vi "rsscope_core_global.vi"() -> ()   [LabVIEW 2018] (continued)
Name"="PCIe Trigger ERRC Unknown Packet", "Data Type"=3, "Command"="TRIG{Trigger}:PCIE:ERRC:UKNP", "Access"=2, "Range Table"="", "Read Callback"="", "Write Callback"="", "Supported Models"="RTO|RTP", "Instrument Options"="K72", "Flags"=0, "Help"="Enables triggering on an unknown packet.\n\nAvailable Repeated Capabilities:\nTrigger: TrigA, TrigB, TrigR\r\n\nRemote-control command(s):\nTRIGger<m>:PCIE:ERRC:UKNP"}, {"Level"=2, "Class Only"=TRUE, "Identifier"="", "Descriptive Name"="EbTb", "Data Type"=0, "Command"="", "Access"=0, "Range Table"="", "Read Callback"="", "Write Callback"="", "Supported Models"="", "Instrument Options"="", "Flags"=0, "Help"="The trigger suffix <m> is always 1 and can be omitted. It selects the trigger event: Only\nthe A-trigger is available for triggering on serial buses."}, {"Level"=3, "Class Only"=FALSE, "Identifier"="RSSCOPE_ATTR_EBTB_TRIGGER_TYPE", "Descriptive Name"="EbTb Trigger Type", "Data Type"=0, "Command"="TRIG{Trigger}:EBTB:TYPE", "Access"=2, "Range Table"="RsScope_rngEbTbTriggerType", "Read Callback"="", "Write Callback"="", "Supported Models"="", "Instrument Options"="", "Flags"=0, "Help"="Selects the type of condition to be triggered on. You can trigger on a certain symbol or enable a specific error condition.\n\nAvailable Repeated Capabilities:\nTrigger: TrigA, TrigB, TrigR\r\n\nRemote-control command(s):\nTRIGger<m>:EBTB:TYPE"}, {"Level"=3, "Class Only"=FALSE, "Identifier"="RSSCOPE_ATTR_EBTB_TRIGGER_CONDITION_TYPE", "Descriptive Name"="EbTb Trigger Condition Type", "Data Type"=0, "Command"="TRIG{Trigger}:EBTB:STYP", "Access"=2, "Range Table"="RsScope_rngTriggerConditionType", "Read Callback"="", "Write Callback"="", "Supported Models"="", "Instrument Options"="", "Flags"=0, "Help"="Selects the type of condition to be triggered on for 8b10b.\n\nAvailable Repeated Capabilities:\nTrigger: TrigA, TrigB, TrigR\r\n\nRemote-control command(s):\nTRIGger<m>:EBTB:STYPe"}, {"Level"=3, "Class Only"=FALSE, "Identifier"="RSSCOPE_ATTR_EBTB_TRIGGER_DISPARITY_ERROR", "Descriptive Name"="EbTb Trigger Disparity Error", "Data Type"=3, "Command"="TRIG{Trigger}:EBTB:DISP", "Access"=2, "Range Table"="", "Read Callback"="", "Write Callback"="", "Supported Models"="", "Instrument Options"="K52", "Flags"=0, "Help"="Defines, if a trigger on a disparity error is activated or not.\n\nAvailable Repeated Capabilities:\nTrigger: TrigA, TrigB, TrigR\r\n\nRemote-control command(s):\nTRIGger<m>:EBTB:DISParityerr"}, {"Level"=3, "Class Only"=FALSE, "Identifier"="RSSCOPE_ATTR_EBTB_TRIGGER_DATA_CHARACTER", "Descriptive Name"="EbTb Trigger Data Character", "Data Type"=0, "Command"="TRIG{Trigger}:EBTB:SYMT", "Access"=2, "Range Table"="RsScope_rngEbTbTriggerDataCharacter", "Read Callback"="", "Write Callback"="", "Supported Models"="", "Instrument Options"="K52", "Flags"=0, "Help"="Selects the data character (Dx.y) or control character to be triggered on. You can specify the value of the data character to be triggered on with RSSCOPE_ATTR_EBTB_TRIGGER_DX_SYMBOL and RSSCOPE_ATTR_EBTB_TRIGGER_DY_SYMBOL.\n\nAvailable Repeated Capabilities:\nTrigger: TrigA, TrigB, TrigR\r\n\nRemote-control command(s):\nTRIGger<m>:EBTB:SYMType"}, {"Level"=3, "Class Only"=FALSE, "Identifier"="RSSCOPE_ATTR_EBTB_TRIGGER_DX_SYMBOL", "Descriptive Name"="EbTb Trigger DX Symbol", "Data Type"=0, "Command"="TRIG{Trigger}:EBTB:DX", "Access"=2, "Range Table"="RsScope_rngEbTbTriggerDXSymbol", "Read Callback"="", "Write Callback"="", "Supported Models"="", "Instrument Options"="K52", "Flags"=0, "Help"="Sets thex value of the data character Dx.y to be triggered on.\n\nAvailable Repeated Capabilities:\nTrigger: TrigA, TrigB, TrigR\r\n\nRemote-control command(s):\nTRIGger<m>:EBTB:DX"}, {"Level"=3, "Class Only"=FALSE, "Identifier"="RSSCOPE_ATTR_EBTB_TRIGGER_DY_SYMBOL", "Descriptive Name"="EbTb Trigger DY Symbol", "Data Type"=0, "Command"="TRIG{Trigger}:EBTB:DY", "Access"=2, "Range Table"="RsScope_rngEbTbTriggerDYSymbol", "Read Callback"="", "Write Callback"="", "Supported Models"="", "Instrument Options"="K52", "Flags"=0, "Help"="Sets the y value of the data character Dx.y to be triggered on.\n\nAvailable Repeated Capabilities:\nTrigger: TrigA, TrigB, TrigR\r\n\nRemote-control command(s):\nTRIGger<m>:EBTB:DY"}, {"Level"=3, "Class Only"=FALSE, "Identifier"="RSSCOPE_ATTR_EBTB_TRIGGER_SYMBOL_FORMAT", "Descriptive Name"="EbTb Trigger Symbol Format", "Data Type"=0, "Command"="TRIG{Trigger}:EBTB:SYMF", "Access"=2, "Range Table"="RsScope_rngEbTbSymbTrgSymbolFormat", "Read Callback"="", "Write Callback"="", "Supported Models"="", "Instrument Options"="K52", "Flags"=0, "Help"="Selects the format of the symbol to be triggerd on, if TRIGger<m>:EBTB:SSTYpe is set to SYMBol.\n\nAvailable Repeated Capabilities:\nTrigger: TrigA, TrigB, TrigR\r\n\nRemote-control command(s):\nTRIGger<m>:EBTB:SYMFormat"}, {"Level"=3, "Class Only"=FALSE, "Identifier"="RSSCOPE_ATTR_EBTB_TRIGGER_EB_PATTERN", "Descriptive Name"="EbTb Trigger EB Pattern", "Data Type"=2, "Command"="TRIG{Trigger}:EBTB:EBPA", "Access"=2, "Range Table"="", "Read Callback"="", "Write Callback"="", "Supported Models"="", "Instrument Options"="K52", "Flags"=0, "Help"="Sets the 8-bit pattern to be triggered on, if TRIGger<m>:EBTB:SYMFormat is set to EB.\n\nAvailable Repeated Capabilities:\nTrigger: TrigA, TrigB, TrigR\r\n\nRemote-control command(s):\nTRIGger<m>:EBTB:EBPA"}, {"Level"=3, "Class Only"=FALSE, "Identifier"="RSSCOPE_ATTR_EBTB_TRIGGER_TB_PATTERN", "Descriptive Name"="EbTb Trigger TB Pattern", "Data Type"=2, "Command"="TRIG{Trigger}:EBTB:TBPA", "Access"=2, "Range Table"="", "Read Callback"="", "Write Callback"="", "Supported Models"="", "Instrument Options"="K52", "Flags"=0, "Help"="Sets the 10-bit pattern to be triggered on, if TRIGger<m>:EBTB:SYMFormat is set to TB.\n\nAvailable Repeated Capabilities:\nTrigger: TrigA, TrigB, TrigR\r\n\nRemote-control command(s):\nTRIGger<m>:EBTB:TBPA"}, {"Level"=3, "Class Only"=FALSE, "Identifier"="RSSCOPE_ATTR_EBTB_TRIGGER_GLITCH_ERROR", "Descriptive Name"="EbTb Trigger Glitch Error", "Data Type"=3, "Command"="TRIG{Trigger}:EBTB:GLIT", "Access"=2, "Range Table"="", "Read Callback"="", "Write Callback"="", "Supported Models"="", "Instrument Options"="K52", "Flags"=0, "Help"="Defines, if a trigger on a glitch error is activated or not.\n\nAvailable Repeated Capabilities:\nTrigger: TrigA, TrigB, TrigR\r\n\nRemote-control command(s):\nTRIGger<m>:EBTB:GLITcherror"}, {"Level"=3, "Class Only"=FALSE, "Identifier"="RSSCOPE_ATTR_EBTB_TRIGGER_SYMBOL_TYPE", "Descriptive Name"="EbTb Trigger Symbol Type", "Data Type"=0, "Command"="TRIG{Trigger}:EBTB:SSTY", "Access"=2, "Range Table"="RsScope_rngEbTbTriggerSymbolType", "Read Callback"="", "Write Callback"="", "Supported Models"="", "Instrument Options"="K52", "Flags"=0, "Help"="Selects the symbol type to be triggered on. You can select a single symbol or an expression (defined series of symbols).\n\nAvailable Repeated Capabilities:\nTrigger: TrigA, TrigB, TrigR\r\n\nRemote-control command(s):\nTRIGger<m>:EBTB:SSTYpe"}, {"Level"=3, "Class Only"=FALSE, "Identifier"="RSSCOPE_ATTR_EBTB_TRIGGER_SYMBOL_EXPRESSION", "Descriptive Name"="EbTb Trigger Symbol Expression", "Data Type"=2, "Command"="TRIG{Trigger}:EBTB:SYME", "Access"=2, "Range Table"="", "Read Callback"="", "Write Callback"="", "Supported Models"="", "Instrument Options"="K52", "Flags"=0, "Help"="Selects the format of the symbol to be triggered on, if TRIGger<m>:EBTB:SSTYpe is set to EXPRession.\n\nAvailable Repeated Capabilities:\nTrigger: TrigA, TrigB, TrigR\r\n\nRemote-control command(s):\nTRIGger<m>:EBTB:SYME"}, {"Level"=3, "Class Only"=FALSE, "Identifier"="RSSCOPE_ATTR_EBTB_TRIGGER_UNKNOWN_ERROR", "Descriptive Name"="EbTb Trigger Unknown Error", "Data Type"=3, "Command"="TRIG{Trigger}:EBTB:UNK", "Access"=2, "Range Table"="", "Read Callback"="", "Write Callback"="", "Supported Models"="", "Instrument Options"="K52", "Flags"=0, "Help"="Defines, if a trigger on a unknown symbol error is activated or not.\n\nAvailable Repeated Capabilities:\nTrigger: TrigA, TrigB, TrigR\r\n\nRemote-control command(s):\nTRIGger<m>:EBTB:UNK"}, {"Level"=2, "Class Only"=TRUE, "Identifier"="", "Descriptive Name"="100BASET1", "Data Type"=0, "Command"="", "Access"=0, "Range Table"="", "Read Callback"="", "Write Callback"="", "Supported Models"="", "Instrument Options"="", "Flags"=0, "Help"="Configures 100BASE-T1 trigger settings.\n\nAttributes in this class require option R&S RTO-K57."}, {"Level"=3, "Class Only"=FALSE, "Identifier"="RSSCOPE_ATTR_100BASE_T1_TRIGGER_TYPE", "Descriptive Name"="100BASE-T1 Trigger Type", "Data Type"=0, "Command"="TRIG{Trigger}:HBTO:TYPE", "Access"=2, "Range Table"="RsScope_rng100BASE_T1FrameType", "Read Callback"="", "Write Callback"="", "Supported Models"="", "Instrument Options"="K57", "Flags"=0, "Help"="Selects the type of frame to be triggered on.\n\nAvailable Repeated Capabilities:\nTrigger: TrigA, TrigB, TrigR\r\n\nRemote-control command(s):\nTRIGger<m>:HBTO:TYPE"}, {"Level"=3, "Class Only"=FALSE, "Identifier"="RSSCOPE_ATTR_100BASE_T1_TRIGGER_DESTINATION_ADDRESS_CONDITION", "Descriptive Name"="100BASE-T1 Trigger Destination Address Condition", "Data Type"=0, "Command"="TRIG{Trigger}:HBTO:DADD:COND", "Access"=2, "Range Table"="rsscope_rngProtocolTriggerCondition", "Read Callback"="", "Write Callback"="", "Supported Models"="", "Instrument Options"="K57", "Flags"=0, "Help"="Sets the condition for the destination address. You can define an exact value or a value range.\n\nAvailable Repeated Capabilities:\nTrigger: TrigA, TrigB, TrigR\r\n\nRemote-control command(s):\nTRIGger<m>:HBTO:DADDress:CONDition"}, {"Level"=3, "Class Only"=FALSE, "Identifier"="RSSCOPE_ATTR_100BASE_T1_TRIGGER_DESTINATION_ADDRESS_MIN", "Descriptive Name"="100BASE-T1 Trigger Destination Address Min", "Data Type"=2, "Command"="TRIG{Trigger}:HBTO:DADD:MIN", "Access"=2, "Range Table"="", "Read Callback"="", "Write Callback"="", "Supported Models"="", "Instrument Options"="K57", "Flags"=0, "Help"="Specifies the destination address bit pattern, or sets the start value of a pattern range.\n\nAvailable Repeated Capabilities:\nTrigger: TrigA, TrigB, TrigR\r\n\nRemote-control command(s):\nTRIGger<m>:HBTO:DADDress:MIN"}, {"Level"=3, "Class Only"=FALSE, "Identifier"="RSSCOPE_ATTR_100BASE_T1_TRIGGER_DESTINATION_ADDRESS_MAX", "Descriptive Name"="100BASE-T1 Trigger Destination Address Max", "Data Type"=2, "Command"="TRIG{Trigger}:HBTO:DADD:MAX", "Access"=2, "Range Table"="", "Read Callback"="", "Write Callback"="", "Supported Models"="", "Instrument Options"="K57", "Flags"=0, "Help"="Sets the end value of the destination address range if the corresponding condition is set to In Range or Out Of Range.\n\nAvailable Repeated Capabilities:\nTrigger: TrigA, TrigB, TrigR\r\n\nRemote-control command(s):\nTRIGger<m>:HBTO:DADDress:MAX"}, {"Level"=3, "Class Only"=FALSE, "Identifier"="RSSCOPE_ATTR_100BASE_T1_TRIGGER_SOURCE_ADDRESS_CONDITION", "Descriptive Name"="100BASE-T1 Trigger Source Address Condition", "Data Type"=0, "Command"="TRIG{Trigger}:HBTO:SADD:COND", "Access"=2, "Range Table"="rsscope_rngProtocolTriggerCondition", "Read Callback"="", "Write Callback"="", "Supported Models"="", "Instrument Options"="K57", "Flags"=0, "Help"="Sets the condition for the source address. You can define an exact value or a value range.\n\nAvailable Repeated Capabilities:\nTrigger: TrigA, TrigB, TrigR\r\n\nRemote-control command(s):\nTRIGger<m>:HBTO:SADDress:CONDition"}, {"Level"=3, "Class Only"=FALSE, "Identifier"="RSSCOPE_ATTR_100BASE_T1_TRIGGER_SOURCE_ADDRESS_MIN", "Descriptive Name"="100BASE-T1 Trigger Source Address Min", "Data Type"=2, "Command"="TRIG{Trigger}:HBTO:SADD:MIN", "Access"=2, "Range Table"="", "Read Callback"="", "Write Callback"="", "Supported Models"="", "Instrument Options"="K57", "Flags"=0, "Help"="Specifies the source address bit pattern, or sets the start value of a pattern range.\n\nAvailable Repeated Capabilities:\nTrigger: TrigA, TrigB, TrigR\r\n\nRemote-control command(s):\nTRIGger<m>:HBTO:SADDress:MIN"}, {"Level"=3, "Class Only"=FALSE, "Identifier"="RSSCOPE_ATTR_100BASE_T1_TRIGGER_SOURCE_ADDRESS_MAX", "Descriptive Name"="100BASE-T1 Trigger Source Address Max", "Data Type"=2, "Command"="TRIG{Trigger}:HBTO:SADD:MAX", "Access"=2, "Range Table"="", "Read Callback"="", "Write Callback"="", "Supported Models"="", "Instrument Options"="K57", "Flags"=0, "Help"="Sets the end value of the source address range if the corresponding condition is set to In Range or Out Of Range.\n\nAvailable Repeated Capabilities:\nTrigger: TrigA, TrigB, TrigR\r\n\nRemote-control command(s):\nTRIGger<m>:HBTO:SADDress:MAX"}, {"Level"=3, "Class Only"=FALSE, "Identifier"="RSSCOPE_ATTR_100BASE_T1_TRIGGER_TYPE_LENGTH_CONDITION", "Descriptive Name"="100BASE-T1 Trigger Type Length Condition", "Data Type"=0, "Command"="TRIG{Trigger}:HBTO:LENG:COND", "Access"=2, "Range Table"="rsscope_rngProtocolTriggerCondition", "Read Callback"="", "Write Callback"="", "Supported Models"="", "Instrument Options"="K57", "Flags"=0, "Help"="Sets the condition for the length / type. You can define an exact value or a value range.\n\nAvailable Repeated Capabilities:\nTrigger: TrigA, TrigB, TrigR\r\n\nRemote-control command(s):\nTRIGger<m>:HBTO:LENGth:CONDition"}, {"Level"=3, "Class Only"=FALSE, "Identifier"="RSSCOPE_ATTR_100BASE_T1_TRIGGER_TYPE_LENGTH_MIN", "Descriptive Name"="100BASE-T1 Trigger Type Length Min", "Data Type"=2, "Command"="TRIG{Trigger}:HBTO:LENG:MIN", "Access"=2, "Range Table"="", "Read Callback"="", "Write Callback"="", "Supported Models"="", "Instrument Options"="", "Flags"=0, "Help"="Specifies the length / type bit pattern, or sets the start value of a pattern range.\n\nAvailable Repeated Capabilities:\nTrigger: TrigA, TrigB, TrigR\r\n\nRemote-control command(s):\nTRIGger<m>:HBTO:LENGth:MIN"}, {"Level"=3, "Class Only"=FALSE, "Identifier"="RSSCOPE_ATTR_100BASE_T1_TRIGGER_TYPE_LENGTH_MAX", "Descriptive Name"="100BASE-T1 Trigger Type Length Max", "Data Type"=2, "Command"="TRIG{Trigger}:HBTO:LENG:MAX", "Access"=2, "Range Table"="", "Read Callback"="", "Write Callback"="", "Supported Models"="", "Instrument Options"="K57", "Flags"=0, "Help"="Sets the end value of the length / type range if the corresponding condition is set to In Range or Out Of Range.\n\nAvailable Repeated Capabilities:\nTrigger: TrigA, TrigB, TrigR\r\n\nRemote-control command(s):\nTRIGger<m>:HBTO:LENGth:MAX"}, {"Level"=3, "Class Only"=FALSE, "Identifier"="RSSCOPE_ATTR_100BASE_T1_TRIGGER_CRC_CONDITION", "Descriptive Name"="100BASE-T1 Trigger CRC Condition", "Data Type"=0, "Command"="TRIG{Trigger}:HBTO:CRC:COND", "Access"=2, "Range Table"="rsscope_rngProtocolTriggerCondition", "Read Callback"="", "Write Callback"="", "Supported Models"="", "Instrument Options"="K57", "Flags"=0, "Help"="Sets the condition for the frame check. You can define an exact value or a value range.\n\nAvailable Repeated Capabilities:\nTrigger: TrigA, TrigB, TrigR\r\n\nRemote-control command(s):\nTRIGger<m>:HBTO:CRC:CONDition"}, {"Level"=3, "Class Only"=FALSE, "Identifier"="RSSCOPE_ATTR_100BASE_T1_TRIGGER_CRC_MIN", "Descriptive Name"="100BASE-T1 Trigger CRC Min", "Data Type"=2, "Command"="TRIG{Trigger}:HBTO:CRC:MIN", "Access"=2, "Range Table"="", "Read Callback"="", "Write Callback"="", "Supported Models"="", "Instrument Options"="K57", "Flags"=0, "Help"="Specifies the frame check bit pattern, or sets the start value of a pattern range.\n\nAvailable Repeated Capabilities:\nTrigger: TrigA, TrigB, TrigR\r\n\nRemote-control command(s):\nTRIGger<m>:HBTO:CRC:MIN"}, {"Level"=3, "Class Only"=FALSE, "Identifier"="RSSCOPE_ATTR_100BASE_T1_TRIGGER_CRC_MAX", "Descriptive Name"="100BASE-T1 Trigger CRC Max", "Data Type"=2, "Command"="TRIG{Trigger}:HBTO:CRC:MAX", "Access"=2, "Range Table"="", "Read Callback"="", "Write Callback"="", "Supported Models"="", "Instrument Options"="K57", "Flags"=0, "Help"="Sets the end value of the frame check range if the corresponding condition is set to In Range or Out Of Range.\n\nAvailable Repeated Capabilities:\nTrigger: TrigA, TrigB, TrigR\r\n\nRemote-control command(s):\nTRIGger<m>:HBTO:CRC:MAX"}, {"Level"=3, "Class Only"=FALSE, "Identifier"="RSSCOPE_ATTR_100BASE_T1_TRIGGER_DATA_CONDITION", "Descriptive Name"="100BASE-T1 Trigger Data Condition", "Data Type"=0, "Command"="TRIG{Trigger}:HBTO:DATA:DCON", "Access"=2, "Range Table"="rsscope_rngProtocolTriggerCondition", "Read Callback"="", "Write Callback"="", "Supported Models"="", "Instrument Options"="K57", "Flags"=0, "Help"="Sets the condition for the data. You can define an exact value or a value range.\n\nAvailable Repeated Capabilities:\nTrigger: TrigA, TrigB, TrigR\r\n\nRemote-control command(s):\nTRIGger<m>:HBTO:DATA:DCONdition"}, {"Level"=3, "Class Only"=FALSE, "Identifier"="RSSCOPE_ATTR_100BASE_T1_TRIGGER_DATA_MIN", "Descriptive Name"="100BASE-T1 Trigger Data Min", "Data Type"=2, "Command"="TRIG{Trigger}:HBTO:DATA:DMIN", "Access"=2, "Range Table"="", "Read Callback"="", "Write Callback"="", "Supported Models"="", "Instrument Options"="K57", "Flags"=0, "Help"="Specifies the data bit pattern, or sets the start value of a pattern range.\n\nAvailable Repeated Capabilities:\nTrigger: TrigA, TrigB, TrigR\r\n\nRemote-control command(s):\nTRIGger<m>:HBTO:DATA:DMIN"}, {"Level"=3, "Class Only"=FALSE, "Identifier"="RSSCOPE_ATTR_100BASE_T1_TRIGGER_DATA_MAX", "Descriptive Name"="100BASE-T1 Trigger Data Max", "Data Type"=2, "Command"="TRIG{Trigger}:HBTO:DATA:DMAX", "Access"=2, "Range Table"="", "Read Callback"="", "Write Callback"="", "Supported Models"="", "Instrument Options"="K57", "Flags"=0, "Help"="Sets the end value of the data range if the corresponding condition is set to In Range or Out Of Range.\n\nAvailable Repeated Capabilities:\nTrigger: TrigA, TrigB, TrigR\r\n\nRemote-control command(s):\nTRIGger<m>:HBTO:DATA:DMAX"}, {"Level"=3, "Class Only"=FALSE, "Identifier"="RSSCOPE_ATTR_100BASE_T1_TRIGGER_INDEX_CONDITION", "Descriptive Name"="100BASE-T1 Trigger Index Condition", "Data Type"=0, "Command"="TRIG{Trigger}:HBTO:DATA:ICON", "Access"=2, "Range Table"="rsscope_rngProtocolTriggerCondition", "Read Callback"="", "Write Callback"="", "Supported Models"="", "Instrument Options"="K57", "Flags"=0, "Help"="Sets the condition for the index. You can define an exact value or a value range.\n\nAvailable Repeated Capabilities:\nTrigger: TrigA, TrigB, TrigR\r\n\nRemote-control command(s):\nTRIGger<m>:HBTO:DATA:ICONdition"}, {"Level"=3, "Class Only"=FALSE, "Identifier"="RSSCOPE_ATTR_100BASE_T1_TRIGGER_INDEX_MIN", "Descriptive Name"="100BASE-T1 Trigger Index Min", "Data Type"=0, "Command"="TRIG{Trigger}:HBTO:DATA:IMIN", "Access"=2, "Range Table"="RsScope_rng100BASE_T1TriggerIndex", "Read Callback"="", "Write Callback"="", "Supported Models"="", "Instrument Options"="K57", "Flags"=0, "Help"="Specifies the index bit pattern, or sets the start value of a pattern range.\n\nAvailable Repeated Capabilities:\nTrigger: TrigA, TrigB, TrigR\r\n\nRemote-control command(s):\nTRIGger<m>:HBTO:DATA:IMIN"}, {"Level"=3, "Class Only"=FALSE, "Identifier"="RSSCOPE_ATTR_100BASE_T1_TRIGGER_INDEX_MAX", "Descriptive Name"="100BASE-T1 Trigger Index Max", "Data Type"=0, "Command"="TRIG{Trigger}:HBTO:DATA:IMAX", "Access"=2, "Range Table"="RsScope_rng100BASE_T1TriggerIndex", "Read Callback"="", "Write Callback"="", "Supported Models"="", "Instrument Options"="K57", "Flags"=0, "Help"="Sets the end value of the index range if the corresponding condition is set to In Range or Out Of Range.\n\nAvailable Repeated Capabilities:\nTrigger: TrigA, TrigB, TrigR\r\n\nRemote-control command(s):\nTRIGger<m>:HBTO:DATA:IMAX"}, {"Level"=3, "Class Only"=FALSE, "Identifier"="RSSCOPE_ATTR_100BASE_T1_TRIGGER_ERROR_PREAMBLE", "Descriptive Name"="100BASE-T1 Trigger Error Preamble", "Data Type"=3, "Command"="TRIG{Trigger}:HBTO:ERR:PRE", "Access"=2, "Range Table"="", "Read Callback"="", "Write Callback"="", "Supported Models"="", "Instrument Options"="K57", "Flags"=0, "Help"="Enables / disables trigger on preamble error.\n\nAvailable Repeated Capabilities:\nTrigger: TrigA, TrigB, TrigR\r\n\nRemote-control command(s):\nTRIGger<m>:HBTO:ERRor:PREamble"}, {"Level"=3, "Class Only"=FALSE, "Identifier"="RSSCOPE_ATTR_100BASE_T1_TRIGGER_ERROR_CRC", "Descriptive Name"="100BASE-T1 Trigger Error CRC", "Data Type"=3, "Command"="TRIG{Trigger}:HBTO:ERR:CRC", "Access"=2, "Range Table"="", "Read Callback"="", "Write Callback"="", "Supported Models"="", "Instrument Options"="K57", "Flags"=0, "Help"="Enables / disables trigger on Cyclic Redundancy Check (CRC) error.\n\nAvailable Repeated Capabilities:\nTrigger: TrigA, TrigB, TrigR\r\n\nRemote-control command(s):\nTRIGger<m>:HBTO:ERRor:CRC"}, {"Level"=3, "Class Only"=FALSE, "Identifier"="RSSCOPE_ATTR_100BASE_T1_TRIGGER_ERROR_SFD", "Descriptive Name"="100BASE-T1 Trigger Error SFD", "Data Type"=3, "Command"="TRIG{Trigger}:HBTO:ERR:SFD", "Access"=2, "Range Table"="", "Read Callback"="", "Write Callback"="", "Supported Models"="", "Instrument Options"="K57", "Flags"=0, "Help"="Enables / disables trigger on start frame delimiter (SFD) error.\n\nAvailable Repeated Capabilities:\nTrigger: TrigA, TrigB, TrigR\r\n\nRemote-control command(s):\nTRIGger<m>:HBTO:ERRor:SFD"}, {"Level"=2, "Class Only"=TRUE, "Identifier"="", "Descriptive Name"="1000BASE-T1", "Data Type"=0, "Command"="", "Access"=0, "Range Table"="", "Read Callback"="", "Write Callback"="", "Supported Models"="", "Instrument Options"="", "Flags"=0, "Help"="Configures 1000BASE-T1 trigger settings with option K58."}, {"Level"=3, "Class Only"=FALSE, "Identifier"="RSSCOPE_ATTR_PROTOCOL_1000BASE_T1_TRIGGER_TYPE", "Descriptive Name"="Protocol 1000BASE-T1 Trigger Type", "Data Type"=0, "Command"="TRIG{Trigger}:TBTO:TYPE", "Access"=2, "Range Table"="RsScope_rngSearch1000BASE_T1Type", "Read Callback"="", "Write Callback"="", "Supported Models"="", "Instrument Options"="K58", "Flags"=0, "Help"="Selects the type of frame to be triggered on.\n\nAvailable Repeated Capabilities:\nTrigger: TrigA, TrigB, TrigR\r\n\nRemote-control command(s):\nTRIGger<m>:TBTO:TYPE"}, {"Level"=3, "Class Only"=FALSE, "Identifier"="RSSCOPE_ATTR_PROTOCOL_1000BASE_T1_TRIGGER_LEVEL", "Descriptive Name"="Protocol 1000BASE-T1 Trigger Level", "Data Type"=1, "Command"="TRIG{Trigger}:TBTO:TRGL", "Access"=2, "Range Table"="RsScope_rngProtocol1000BASET1TriggerLevel", "Read Callback"="", "Write Callback"="", "Supported Models"="", "Instrument Options"="K58", "Flags"=0, "Help"="Sets the trigger level.\n\nAvailable Repeated Capabilities:\nTrigger: TrigA, TrigB, TrigR\r\n\nRemote-control command(s):\nTRIGger<m>:TBTO:TRGLevel"}, {"Level"=3, "Class Only"=FALSE, "Identifier"="RSSCOPE_ATTR_PROTOCOL_1000BASE_T1_TRIGGER_DESTINATION_ADDRESS_CONDITION", "Descriptive Name"="Protocol 1000BASE-T1 Trigger Destination Address Condition", "Data Type"=0, "Command"="TRIG{Trigger}:TBTO:DADD:COND", "Access"=2, "Range Table"="rsscope_rngProtocolTriggerConditionStrict", "Read Callback"="", "Write Callback"="", "Supported Models"="", "Instrument Options"="K58", "Flags"=0, "Help"="Sets the condition for the destination address. You can define an exact value or a value range.\n\nAvailable Repeated Capabilities:\nTrigger: TrigA, TrigB, TrigR\r\n\nRemote-control command(s):\nTRIGger<m>:TBTO:DADDress:CONDition"}, {"Level"=3, "Class Only"=FALSE, "Identifier"="RSSCOPE_ATTR_PROTOCOL_1000BASE_T1_TRIGGER_DESTINATION_ADDRESS_MIN", "Descriptive Name"="Protocol 1000BASE-T1 Trigger Destination Address Min", "Data Type"=2, "Command"="TRIG{Trigger}:TBTO:DADD:MIN", "Access"=2, "Range Table"="", "Read Callback"="", "Write Callback"="", "Supported Models"="", "Instrument Options"="K58", "Flags"=0, "Help"="Specifies the destination address bit pattern, or sets the start value of a pattern range. The string parameter accepts the bit value X (do not care).\n\nAvailable Repeated Capabilities:\nTrigger: TrigA, TrigB, TrigR\r\n\nRemote-control command(s):\nTRIGger<m>:TBTO:DADDress:MIN"}, {"Level"=3, "Class Only"=FALSE, "Identifier"="RSSCOPE_ATTR_PROTOCOL_1000BASE_T1_TRIGGER_DESTINATION_ADDRESS_MAX", "Descriptive Name"="Protocol 1000BASE-T1 Trigger Destination Address Max", "Data Type"=2, "Command"="TRIG{Trigger}:TBTO:DADD:MAX", "Access"=2, "Range Table"="", "Read Callback"="", "Write Callback"="", "Supported Models"="", "Instrument Options"="K58", "Flags"=0, "Help"="Sets the end value of the destination address range if RSSCOPE_ATTR_PROTOCOL_1000BASE_T1_TRIGGER_DESTINATION_ADDRESS_CONDITION is set to In Range or Out Of Range. The string parameter accepts the bit value X (do not care).\n\nAvailable Repeated Capabilities:\nTrigger: TrigA, TrigB, TrigR\r\n\nRemote-control command(s):\nTRIGger<m>:TBTO:DADDress:MAX"}, {"Level"=3, "Class Only"=FALSE, "Identifier"="RSSCOPE_ATTR_PROTOCOL_1000BASE_T1_TRIGGER_SOURCE_ADDRESS_CONDITION", "Descriptive Name"="Protocol 1000BASE-T1 Trigger Source Address Condition", "Data Type"=0, "Command"="TRIG{Trigger}:TBTO:SADD:COND", "Access"=2, "Range Table"="rsscope_rngProtocolTriggerConditionStrict", "Read Callback"="", "Write Callback"="", "Supported Models"="", "Instrument Options"="K58", "Flags"=0, "Help"="Sets the condition for the source address. You can define an exact value or a value range.\n\nAvailable Repeated Capabilities:\nTrigger: TrigA, TrigB, TrigR\r\n\nRemote-control command(s):\nTRIGger<m>:TBTO:SADDress:CONDition"}, {"Level"=3, "Class Only"=FALSE, "Identifier"="RSSCOPE_ATTR_PROTOCOL_1000BASE_T1_TRIGGER_SOURCE_ADDRESS_MIN", "Descriptive Name"="Protocol 1000BASE-T1 Trigger Source Address Min", "Data Type"=2, "Command"="TRIG{Trigger}:TBTO:SADD:MIN", "Access"=2, "Range Table"="", "Read Callback"="", "Write Callback"="", "Supported Models"="", "Instrument Options"="K58", "Flags"=0, "Help"="Specifies the source address bit pattern, or sets the start value of a pattern range. The string parameter accepts the bit value X (do not care).\n\nAvailable Repeated Capabilities:\nTrigger: TrigA, TrigB, TrigR\r\n\nRemote-control command(s):\nTRIGger<m>:TBTO:SADDress:MIN"}, {"Level"=3, "Class Only"=FALSE, "Identifier"="RSSCOPE_ATTR_PROTOCOL_1000BASE_T1_TRIGGER_SOURCE_ADDRESS_MAX", "Descriptive Name"="Protocol 1000BASE-T1 Trigger Source Address Max", "Data Type"=2, "Command"="TRIG{Trigger}:TBTO:SADD:MAX", "Access"=2, "Range Table"="", "Read Callback"="", "Write Callback"="", "Supported Models"="", "Instrument Options"="K58", "Flags"=0, "Help"="Sets the end value of the source address range, if RSSCOPE_ATTR_PROTOCOL_1000BASE_T1_TRIGGER_SOURCE_ADDRESS_CONDITION is set to In Range or Out Of Range. The string parameter accepts the bit value X (do not care).\n\nAvailable Repeated Capabilities:\nTrigger: TrigA, TrigB, TrigR\r\n\nRemote-control command(s):\nTRIGger<m>:TBTO:SADDress:MAX"}, {"Level"=3, "Class Only"=FALSE, "Identifier"="RSSCOPE_ATTR_PROTOCOL_1000BASE_T1_TRIGGER_LENGTH_TYPE_CONDITION", "Descriptive Name"="Protocol 1000BASE-T1 Trigger Length Type Condition", "Data Type"=0, "Command"="TRIG{Trigger}:TBTO:LENG:COND", "Access"=2, "Range Table"="rsscope_rngProtocolTriggerConditionStrict", "Read Callback"="", "Write Callback"="", "Supported Models"="", "Instrument Options"="K58", "Flags"=0, "Help"="Sets the condition for the length / type. You can define an exact value or a value range.\n\nAvailable Repeated Capabilities:\nTrigger: TrigA, TrigB, TrigR\r\n\nRemote-control command(s):\nTRIGger<m>:TBTO:LENGth:CONDition"}, {"Level"=3, "Class Only"=FALSE, "Identifier"="RSSCOPE_ATTR_PROTOCOL_1000BASE_T1_TRIGGER_LENGTH_TYPE_MIN", "Descriptive Name"="Protocol 1000BASE-T1 Trigger Length Type Min", "Data Type"=2, "Command"="TRIG{Trigger}:TBTO:LENG:MIN", "Access"=2, "Range Table"="", "Read Callback"="", "Write Callback"="", "Supported Models"="", "Instrument Options"="K58", "Flags"=0, "Help"="Specifies the length / type bit pattern, or sets the start value of a pattern range. The string parameter accepts the bit value X (do not care).\n\nAvailable Repeated Capabilities:\nTrigger: TrigA, TrigB, TrigR\r\n\nRemote-control command(s):\nTRIGger<m>:TBTO:LENGth:MIN"}, {"Level"=3, "Class Only"=FALSE, "Identifier"="RSSCOPE_ATTR_PROTOCOL_1000BASE_T1_TRIGGER_LENGTH_TYPE_MAX", "Descriptive Name"="Protocol 1000BASE-T1 Trigger Length Type Max", "Data Type"=2, "Command"="TRIG{Trigger}:TBTO:LENG:MAX", "Access"=2, "Range Table"="", "Read Callback"="", "Write Callback"="", "Supported Models"="", "Instrument Options"="K58", "Flags"=0, "Help"="Sets the end value of the length / type range if RSSCOPE_ATTR_PROTOCOL_1000BASE_T1_TRIGGER_LENGTH_TYPE_CONDITION is set to In Range or Out Of Range. The string parameter accepts the bit value X (do not care).\n\nAvailable Repeated Capabilities:\nTrigger: TrigA, TrigB, TrigR\r\n\nRemote-control command(s):\nTRIGger<m>:TBTO:LENGth:MAX"}, {"Level"=3, "Class Only"=FALSE, "Identifier"="RSSCOPE_ATTR_PROTOCOL_1000BASE_T1_TRIGGER_FRAME_CHECK_CRC_CONDITION", "Descriptive Name"="Protocol 1000BASE-T1 Trigger Frame Check CRC Condition", "Data Type"=0, "Command"="TRIG{Trigger}:TBTO:CRC:COND", "Access"=2, "Range Table"="rsscope_rngProtocolTriggerConditionStrict", "Read Callback"="", "Write Callback"="", "Supported Models"="", "Instrument Options"="K58", "Flags"=0, "Help"="Sets the condition for the frame check. You can define an exact value or a value range.\n\nAvailable Repeated Capabilities:\nTrigger: TrigA, TrigB, TrigR\r\n\nRemote-control command(s):\nTRIGger<m>:TBTO:CRC:CONDition"}, {"Level"=3, "Class Only"=FALSE, "Identifier"="RSSCOPE_ATTR_PROTOCOL_1000BASE_T1_TRIGGER_FRAME_CHECK_CRC_MIN", "Descriptive Name"="Protocol 1000BASE-T1 Trigger Frame Check CRC Min", "Data Type"=2, "Command"="TRIG{Trigger}:TBTO:CRC:MIN", "Access"=2, "Range Table"="", "Read Callback"="", "Write Callback"="", "Supported Models"="", "Instrument Options"="K58", "Flags"=0, "Help"="Specifies the frame check bit pattern, or sets the start value of a pattern range. The string parameter accepts the bit value X (do not care).\n\nAvailable Repeated Capabilities:\nTrigger: TrigA, TrigB, TrigR\r\n\nRemote-control command(s):\nTRIGger<m>:TBTO:CRC:MIN"}, {"Level"=3, "Class Only"=FALSE, "Identifier"="RSSCOPE_ATTR_PROTOCOL_1000BASE_T1_TRIGGER_FRAME_CHECK_CRC_MAX", "Descriptive Name"="Protocol 1000BASE-T1 Trigger Frame Check CRC Max", "Data Type"=2, "Command"="TRIG{Trigger}:TBTO:CRC:MAX", "Access"=2, "Range Table"="", "Read Callback"="", "Write Callback"="", "Supported Models"="", "Instrument Options"="K58", "Flags"=0, "Help"="Sets the end value of the frame check range if RSSCOPE_ATTR_PROTOCOL_1000BASE_T1_TRIGGER_FRAME_CHECK_CRC_CONDITION is set to In Range or Out Of Range. The string parameter accepts the bit value X (do not care).\n\nAvailable Repeated Capabilities:\nTrigger: TrigA, TrigB, TrigR\r\n\nRemote-control command(s):\nTRIGger<m>:TBTO:CRC:MAX"}, {"Level"=3, "Class Only"=FALSE, "Identifier"="RSSCOPE_ATTR_PROTOCOL_1000BASE_T1_TRIGGER_DATA_CONDITION", "Descriptive Name"="Protocol 1000BASE-T1 Trigger Data Condition", "Data Type"=0, "Command"="TRIG{Trigger}:TBTO:DATA:DCON", "Access"=2, "Range Table"="rsscope_rngProtocolTriggerConditionStrict", "Read Callback"="", "Write Callback"="", "Supported Models"="", "Instrument Options"="K58", "Flags"=0, "Help"="Sets the condition for the data. You can define an exact value or a value range.\n\nAvailable Repeated Capabilities:\nTrigger: TrigA, TrigB, TrigR\r\n\nRemote-control command(s):\nTRIGger<m>:TBTO:DATA:DCONdition"}, {"Level"=3, "Class Only"=FALSE, "Identifier"="RSSCOPE_ATTR_PROTOCOL_1000BASE_T1_TRIGGER_DATA_MIN", "Descriptive Name"="Protocol 1000BASE-T1 Trigger Data Min", "Data Type"=2, "Command"="TRIG{Trigger}:TBTO:DATA:DMIN", "Access"=2, "Range Table"="", "Read Callback"="", "Write Callback"="", "Supported Models"="", "Instrument Options"="K58", "Flags"=0, "Help"="Specifies the data bit pattern, or sets the start value of a pattern range. The string parameter accepts the bit value X (do not care).\n\nAvailable Repeated Capabilities:\nTrigger: TrigA, TrigB, TrigR\r\n\nRemote-control command(s):\nTRIGger<m>:TBTO:DATA:DMIN"}, {"Level"=3, "Class Only"=FALSE, "Identifier"="RSSCOPE_ATTR_PROTOCOL_1000BASE_T1_TRIGGER_DATA_MAX", "Descriptive Name"="Protocol 1000BASE-T1 Trigger Data Max", "Data Type"=2, "Command"="TRIG{Trigger}:TBTO:DATA:DMAX", "Access"=2, "Range Table"="", "Read Callback"="", "Write Callback"="", "Supported Models"="", "Instrument Options"="K58", "Flags"=0, "Help"="Sets the end value of the data range if RSSCOPE_ATTR_PROTOCOL_1000BASE_T1_TRIGGER_DATA_CONDITION is set to In Range or Out Of Range. The string parameter accepts the bit value X (do not care).\n\nAvailable Repeated Capabilities:\nTrigger: TrigA, TrigB, TrigR\r\n\nRemote-control command(s):\nTRIGger<m>:TBTO:DATA:DMAX"}, {"Level"=3, "Class Only"=FALSE, "Identifier"="RSSCOPE_ATTR_PROTOCOL_1000BASE_T1_TRIGGER_INDEX_CONDITION", "Descriptive Name"="Protocol 1000BASE-T1 Trigger Index Condition", "Data Type"=0, "Command"="TRIG{Trigger}:TBTO:DATA:ICON", "Access"=2, "Range Table"="rsscope_rngProtocolTriggerConditionStrict", "Read Callback"="", "Write Callback"="", "Supported Models"="", "Instrument Options"="K58", "Flags"=0, "Help"="Sets the condition for the index. You can define an exact value or a value range.\n\nAvailable Repeated Capabilities:\nTrigger: TrigA, TrigB, TrigR\r\n\nRemote-control command(s):\nTRIGger<m>:TBTO:DATA:ICONdition"}, {"Level"=3, "Class Only"=FALSE, "Identifier"="RSSCOPE_ATTR_PROTOCOL_1000BASE_T1_TRIGGER_INDEX_MIN", "Descriptive Name"="Protocol 1000BASE-T1 Trigger Index Min", "Data Type"=0, "Command"="TRIG{Trigger}:TBTO:DATA:IMIN", "Access"=2, "Range Table"="RsScope_rng1000BASET1Index", "Read Callback"="", "Write Callback"="", "Supported Models"="", "Instrument Options"="K58", "Flags"=0, "Help"="Specifies the index bit pattern, or sets the start value of a pattern range. In binary format, use the following characters: 1; 0; or X (do not care).\n\nAvailable Repeated Capabilities:\nTrigger: TrigA, TrigB, TrigR\r\n\nRemote-control command(s):\nTRIGger<m>:TBTO:DATA:IMIN"}, {"Level"=3, "Class Only"=FALSE, "Identifier"="RSSCOPE_ATTR_PROTOCOL_1000BASE_T1_TRIGGER_INDEX_MAX", "Descriptive Name"="Protocol 1000BASE-T1 Trigger Index Max", "Data Type"=0, "Command"="TRIG{Trigger}:TBTO:DATA:IMAX", "Access"=2, "Range Table"="RsScope_rng1000BASET1Index", "Read Callback"="", "Write Callback"="", "Supported Models"="", "Instrument Options"="K58", "Flags"=0, "Help"="Sets the end value of the index range if RSSCOPE_ATTR_PROTOCOL_1000BASE_T1_TRIGGER_INDEX_CONDITION is set to In Range or Out Of Range. In binary format, use the following characters: 1; 0; or X (do not care).\n\nAvailable Repeated Capabilities:\nTrigger: TrigA, TrigB, TrigR\r\n\nRemote-control command(s):\nTRIGger<m>:TBTO:DATA:IMAX"}, {"Level"=3, "Class Only"=FALSE, "Identifier"="RSSCOPE_ATTR_PROTOCOL_1000BASE_T1_TRIGGER_ERROR_RS_FEC", "Descriptive Name"="Protocol 1000BASE-T1 Trigger Error RS-FEC", "Data Type"=3, "Command"="TRIG{Trigger}:TBTO:ERR:FEC", "Access"=2, "Range Table"="", "Read Callback"="", "Write Callback"="", "Supported Models"="", "Instrument Options"="K58", "Flags"=0, "Help"="Enables triggering, if more than 22 RS-FEC errors are detected.\n\nAvailable Repeated Capabilities:\nTrigger: TrigA, TrigB, TrigR\r\n\nRemote-control command(s):\nTRIGger<m>:TBTO:ERRor:FEC"}, {"Level"=3, "Class Only"=FALSE, "Identifier"="RSSCOPE_ATTR_PROTOCOL_1000BASE_T1_TRIGGER_ERROR_CRC", "Descriptive Name"="Protocol 1000BASE-T1 Trigger Error CRC", "Data Type"=3, "Command"="TRIG{Trigger}:TBTO:ERR:CRC", "Access"=2, "Range Table"="", "Read Callback"="", "Write Callback"="", "Supported Models"="", "Instrument Options"="K58", "Flags"=0, "Help"="Enables triggering on cyclic redundancy check (CRC) error.\n\nAvailable Repeated Capabilities:\nTrigger: TrigA, TrigB, TrigR\r\n\nRemote-control command(s):\nTRIGger<m>:TBTO:ERRor:CRC"}, {"Level"=3, "Class Only"=FALSE, "Identifier"="RSSCOPE_ATTR_PROTOCOL_1000BASE_T1_TRIGGER_ERROR_OUT_OF_RANGE", "Descriptive Name"="Protocol 1000BASE-T1 Trigger Error Out Of Range", "Data Type"=3, "Command"="TRIG{Trigger}:TBTO:ERR:OOR", "Access"=2, "Range Table"="", "Read Callback"="", "Write Callback"="", "Supported Models"="", "Instrument Options"="K58", "Flags"=0, "Help"="Enables triggering if values are out of range (OOR). For example, a preamble error, or invalid symbols in control blocks.\n\nAvailable Repeated Capabilities:\nTrigger: TrigA, TrigB, TrigR\r\n\nRemote-control command(s):\nTRIGger<m>:TBTO:ERRor:OOR"}, {"Level"=3, "Class Only"=FALSE, "Identifier"="RSSCOPE_ATTR_PROTOCOL_1000BASE_T1_TRIGGER_ERROR_ZERO_TERNARY_SYMBOL", "Descriptive Name"="Protocol 1000BASE-T1 Trigger Error Zero Ternary Symbol", "Data Type"=3, "Command"="TRIG{Trigger}:TBTO:ERR:ZERO", "Access"=2, "Range Table"="", "Read Callback"="", "Write Callback"="", "Supported Models"="", "Instrument Options"="K58", "Flags"=0, "Help"="Enables triggering, if a zero ternary symbol pair (0-0) is detected.\n\nAvailable Repeated Capabilities:\nTrigger: TrigA, TrigB, TrigR\r\n\nRemote-control command(s):\nTRIGger<m>:TBTO:ERRor:ZERO"}, {"Level"=1, "Class Only"=TRUE, "Identifier"="", "Descriptive Name"="Waveform Acquisition", "Data Type"=0, "Command"="", "Access"=0, "Range Table"="", "Read Callback"="", "Write Callback"="", "Supported Models"="", "Instrument Options"="", "Flags"=0, "Help"="Attributes that configure the waveform measurement."}, {"Level"=2, "Class Only"=FALSE, "Identifier"="RSSCOPE_ATTR_RUN_SINGLE", "Descriptive Name"="Run Single", "Data Type"=4, "Command"="SING", "Access"=1, "Range Table"="", "Read Callback"="", "Write Callback"="", "Supported Models"="", "Instrument Options"="", "Flags"=1, "Help"="Starts a defined number of acquisition cycles and waits for the acquisition to be finished. For settings of sweep count see RSSCOPE_ATTR_NUM_AVERAGES.\n\nAvailable Repeated Capabilities:\nNone\n\nRemote-control command(s):\nSINGle"}, {"Level"=2, "Class Only"=FALSE, "Identifier"="RSSCOPE_ATTR_RUN_SINGLE_WITHOUT_WAIT", "Descriptive Name"="Run Single Without Wait", "Data Type"=4, "Command"="SING", "Access"=1, "Range Table"="", "Read Callback"="", "Write Callback"="", "Supported Models"="", "Instrument Options"="", "Flags"=0, "Help"="Starts a defined number of acquisition cycles. For settings of sweep count see RSSCOPE_ATTR_NUM_AVERAGES. Does not wait for operation to complete.\n\nAvailable Repeated Capabilities:\nNone\n\nRemote-control command(s):\nSINGle"}, {"Level"=2, "Class Only"=FALSE, "Identifier"="RSSCOPE_ATTR_RUN_CONTINUOUS", "Descriptive Name"="Run Continuous", "Data Type"=4, "Command"="RUN", "Access"=1, "Range Table"="", "Read Callback"="", "Write Callback"="", "Supported Models"="", "Instrument Options"="", "Flags"=0, "Help"="Starts the continuous acquisition.\n\nAvailable Repeated Capabilities:\nNone\n\nRemote-control command(s):\nRUN"}, {"Level"=2, "Class Only"=FALSE, "Identifier"="RSSCOPE_ATTR_STOP", "Descriptive Name"="Stop", "Data Type"=4, "Command"="STOP", "Access"=1, "Range Table"="", "Read Callback"="", "Write Callback"="", "Supported Models"="", "Instrument Options"="", "Flags"=0, "Help"="Stops the running acquistion.\n\nAvailable Repeated Capabilities:\nNone\n\nRemote-control command(s):\nSTOP"}, {"Level"=2, "Class Only"=FALSE, "Identifier"="RSSCOPE_ATTR_FORCE", "Descriptive Name"="Force", "Data Type"=4, "Command"="TRIG:FORC", "Access"=1, "Range Table"="", "Read Callback"="", "Write Callback"="", "Supported Models"="", "Instrument Options"="", "Flags"=0, "Help"="If the acquisition is running in normal mode and no valid trigger occurs, forcing the trigger provokes an immediate single acquisition. Thus you can confirm that a signal is available and use the waveform display to determine how to trigger on it.\n\nAvailable Repeated Capabilities:\nNone\n\nRemote-control command(s):\nTRIGger<m>:FORCe"}, {"Level"=2, "Class Only"=FALSE, "Identifier"="RSSCOPE_ATTR_SEND_SW_TRIGGER", "Descriptive Name"="Send SW Trigger", "Data Type"=4, "Command"="*TRG", "Access"=1, "Range Table"="", "Read Callback"="", "Write Callback"="", "Supported Models"="", "Instrument Options"="", "Flags"=0, "Help"="Triggers 
